vi "Create New System Definition.vi"(8 "error in":errorcluster, 10 "OS (Windows)":string="Windows", 11 "System Definition Name":string) -> (0 "error out":errorcluster, 3 "System Definition Path":path)   [LabVIEW 2020]
uses:
  NationalInstruments.VeriStand.SystemDefinitionAPI
  niveristand-custom-device-testing-tools/VeriStandTestUtilities/VeriStandTestUtilities.lvlib
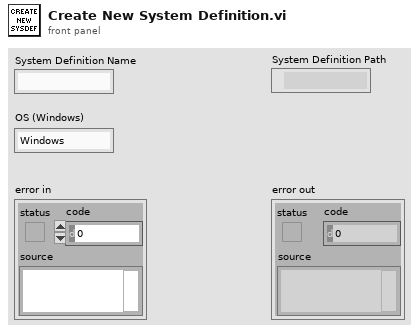
[diagram p1: front panel]
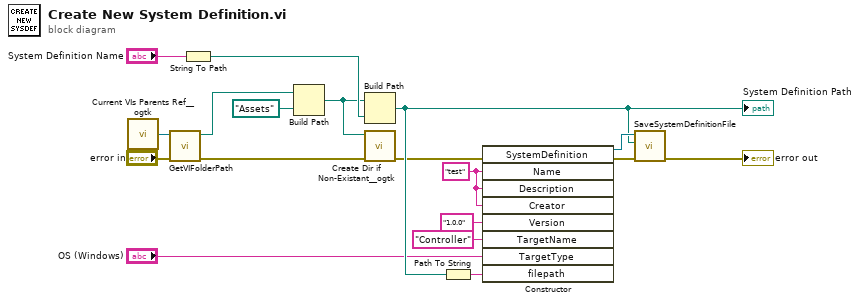
[diagram p0: block diagram]
diagram:
  w13 = "test" ("Name")
  n1 = call <userlib>:"Current VIs Parents Ref__ogtk.vi"() -> ("Calling VI's Reference"=w18:refnum<vi>)  [unwired: 2 in]
  n2 = call "GetVIFolderPath.vi"("error in (no error)"="error in", "VI Reference in"=w18) -> ("error out"=w3:errorcluster, "VI Folder Path out"=w16:path)  [unwired: 8 in]
  n3 = String To Path(string="System Definition Name") -> (path=w5:path)
  n4 = Build Path(base path=w16, name or relative path=path "Assets" ("Absolute or Relative Path")) -> (appended path=w2:path)
  n5 = Build Path(base path=w2, name or relative path=w5) -> (appended path=w8:path)
  "System Definition Path" <- w8
  n6 = call <userlib>:"Create Dir if Non-Existant__ogtk.vi"("error in (no error)"=w3, "Directory Path"=w2) -> ("error out"=w1:errorcluster)  [unwired: 7 in, 2 out]
  n7 = Path To String(path=w8) -> (string=w14:string)
  n8 = constructor class="SystemDefinition"(error in=w1, "Name"=w13, "Description"=w13, "Creator"=w13, "Version"="1.0.0", "TargetName"="Controller", "TargetType"="OS (Windows)", "filepath"=w14) -> (reference out=w9:refnum<k24>, error out=w10:errorcluster)  [unwired: 2 in, 8 out]
  n9 = call "SaveSystemDefinitionFile.vi"("error in (no error)"=w10, "System Definition File in"=w8, "System Definition Reference in"=w9) -> ("error out"=→"error out":errorcluster)  [unwired: 7 in, 1 out]
